vi "Parker Stepper Client.vi"(2 "Point #":i32, 4 "Parameters":dbl[](array[numeric]) format="%.2f", 5 "Port":refnum<visa-resource-name>) -> (0 "Stop":bool, 1 "Data Out":dbl[](array[numeric]) format="%.2f")   [LabVIEW 2020]
panel:
  out "?":cluster{dbl[]}[](graph)
  out "messages":string
  in  "host:station":string="Data5Mac.magnet.fsu.edu:Parker Stepper Control"
  out "StationVIReference":refnum<vi>
  out "error out":errorcluster
  in  "error in (no error)":errorcluster
  out "plot name":string
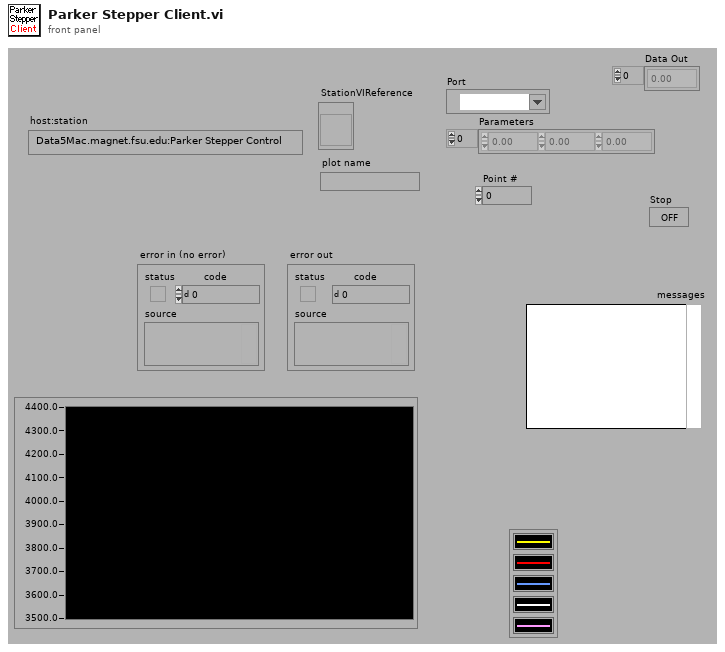
[diagram p1: front panel]
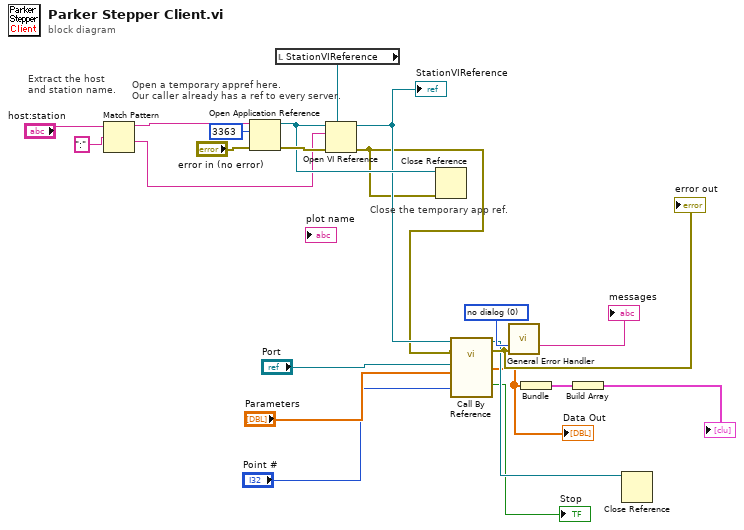
[diagram p0: block diagram]
diagram:
  w16 = u16 0 items=["no dialog", "OK message", "continue or stop message"] ("type of dialog (OK msg:1)")
  # "Open a temporary appref here.\nOur caller already has a ref to every server."
  # "Close the temporary app ref."
  # "Extract the host\nand station name."
  n1 = Match Pattern(string="host:station", regular expression=":") -> (before substring=w8:string, after substring=w7:string)  [unwired: 1 in, 2 out]
  n2 = Open Application Reference(8:"error in (no error)", 10:u32 3363 ("port number (3363)"), 11:w8) -> (0:w18:errorcluster, 3:w17:refnum<vi>)  [unwired: 1 in]
  n3 = local read "StationVIReference"() -> (w19:refnum<vi>)
  n4 = Open VI Reference(type specifier VI Refnum (for type only)=w19, application reference (local)=w17, vi path=w7, error in (no error)=w18) -> (vi reference=w15:refnum<vi>, error out=w14:errorcluster)  [unwired: 2 in]
  "StationVIReference" <- w15
  n5 = Close Reference(reference=w17, error in (no error)=w14) -> ()  [unwired: 1 out]
  n6 = call-by-ref "?"(reference=w15, error in=w14, "Point #"="Point #", "Parameters"="Parameters", "Instrument Address"="Port") -> (reference out=w9:refnum<vi>, error out=w10:errorcluster, "Stop"=→"Stop":bool, "Data Out"=w3:dbl[])  [unwired: 1 in]
  "error out" <- w10
  "Data Out" <- w3
  n7 = call <vilib>:"General Error Handler.vi"("type of dialog (OK msg:1)"=w16, "error in (no error)"=w10) -> ("message"=→"messages":string)  [unwired: 9 in, 4 out]
  n8 = Bundle("Data Out"=w3) -> (w12:cluster{"Data Out":dbl[]})  [unwired: 1 in]
  n9 = Build Array(w12) -> (→"?":cluster{"Data Out":dbl[]}[])
  n10 = Close Reference(reference=w9) -> ()  [unwired: 1 in, 1 out]
